vi "launch-fi-engine.vi"(8 "error in (no error)":errorcluster, 11 "fi in":refnum<class "bFrameIO.lvclass">) -> (0 "error out":errorcluster, 3 "fi out":refnum<class "bFrameIO.lvclass">)   [LabVIEW 2015, in "bFrameIO.lvclass"]
uses:
  bFrameIO.lvclass
  bFrameIO.lvclass/bFrameIO.ctl
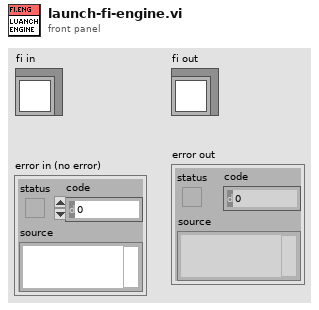
[diagram p1: front panel]
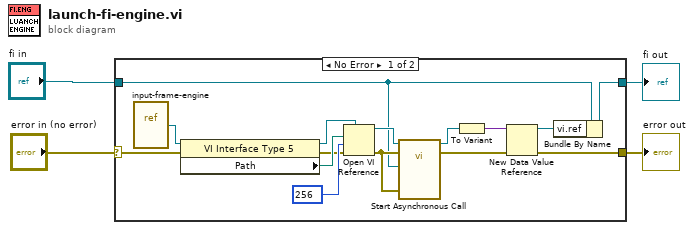
[diagram p0: block diagram]
diagram:
  n1 = case shown="No Error" "error in (no error)" {
    selector: "error in (no error)" -> [w13 w21]
    tunnel: [w10 w21] -> w3
    tunnel: [w6 w20] -> w1
    tunnel: "fi in" -> [w7 w20]
    frame No Error {
      n2 = vi-ref "input-frame-engine.vi"() -> (w19:refnum<vi>)
      n3 = property class="VI Interface Type 5"(reference=w19, error in=w13) -> (reference out=w18:refnum<vi>, error out=w12:errorcluster, "Path"=w17:path)
      n4 = Open VI Reference(type specifier VI Refnum (for type only)=w18, vi path=w17, options=256, error in (no error)=w12) -> (vi reference=w15:refnum<vi>, error out=w14:errorcluster)  [unwired: 2 in]
      n5 = call-by-ref "Start Asynchronous Call"(reference=w15, error in=w14, 8:"error in (no error)"=w14, "dbc in"=w7) -> (reference out=w8:refnum<vi>, error out=w11:errorcluster)  [unwired: 8 in, 2 out]
      n6 = To Variant(anything=w8) -> (Variant=w9:variant)
      n7 = New Data Value Reference(data value=w9, error in=w11) -> (data value reference=w5:refnum<data-value>, error out=w10:errorcluster)
      n8 = Bundle By Name(cluster=w7, "vi.ref"=w5) -> (w6:refnum<class "bFrameIO.lvclass">)
    }
    frame Error {
    }
  }
  "error out" <- w3
  "fi out" <- w1
